vi "Get Index File Path.vi"(8 "error in (no error)":errorcluster, 10 "Project or Class Path":path, 11 "Indexing Test Finder in":refnum<class "Indexing Test Finder.lvclass">) -> (0 "error out":errorcluster, 2 "Index File Path":path, 3 "Indexing Test Finder out":refnum<class "Indexing Test Finder.lvclass">)   [LabVIEW 2020, in "Indexing Test Finder.lvclass"]
uses:
  Indexing Test Finder.lvclass
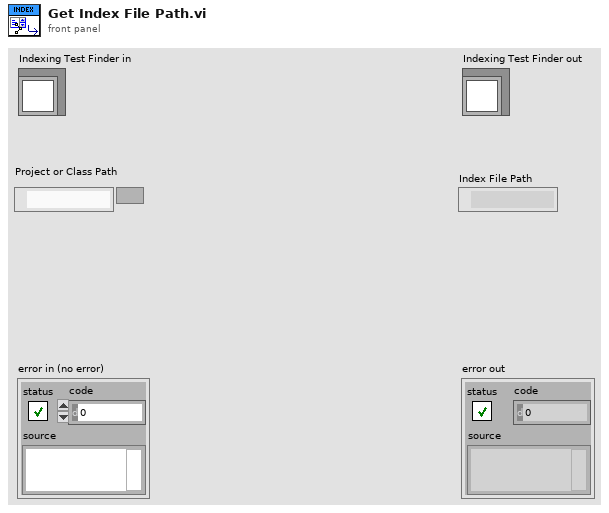
[diagram p1: front panel]
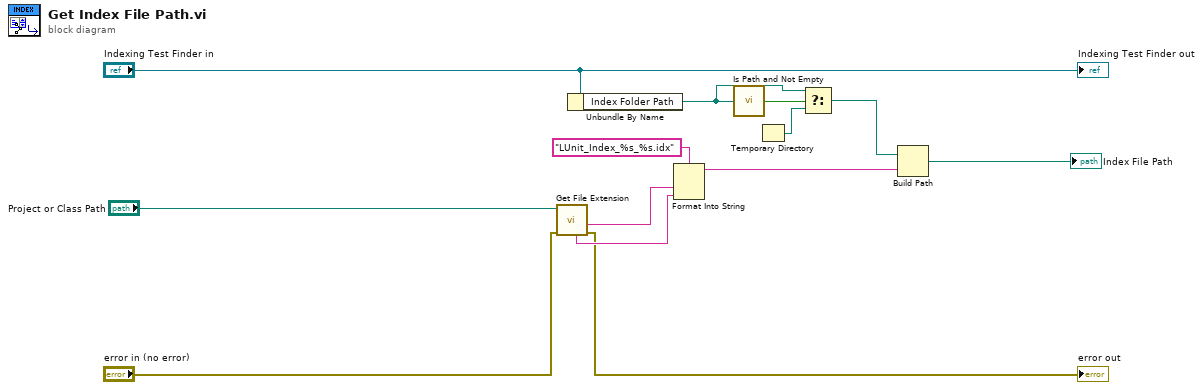
[diagram p0: block diagram]
diagram:
  n1 = call <vilib>:"Get File Extension.vi"("error in (no error)"="error in (no error)", "file"="Project or Class Path") -> ("error out"=→"error out":errorcluster, "filename without extension"=w8:string, "unmodified file extension"=w7:string)  [unwired: 5 in, 2 out]
  n2 = Unbundle By Name("Indexing Test Finder in") -> ("Index Folder Path"=w4:path)
  n3 = Format Into String(format string="LUnit_Index_%s_%s.idx", w8, w7) -> (resulting string=w11:string)  [unwired: 2 in, 1 out]
  n4 = call <vilib>:"Is Path and Not Empty.vi"("path"=w4) -> ("Is Path and Not Empty?"=w5:bool)  [unwired: 4 in]
  n5 = Temporary Directory() -> (w2:path)
  n6 = Select(t=w4, s=w5, f=w2) -> (s? t:f=w3:path)
  n7 = Build Path(base path=w3, name or relative path=w11) -> (appended path=→"Index File Path":path)
  "Indexing Test Finder out" <- "Indexing Test Finder in"
